vi "server.vi"() -> ()   [LabVIEW 2016]
uses:
  <vilib>/NI/NI JSONRPC Server Framework/Classes/Server/Send Request (Sync).vi
  <vilib>/NI/NI JSONRPC Server Framework/Classes/Server/JSONRPC Server.lvclass
panel:
  in  "stop server":bool
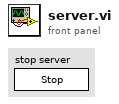
[diagram p1: front panel]
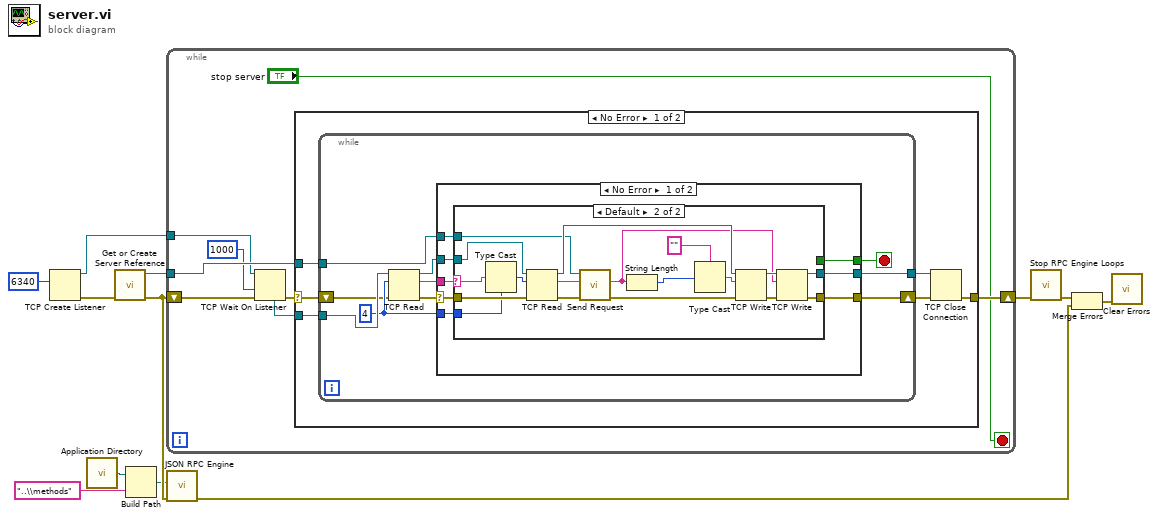
[diagram p0: block diagram]
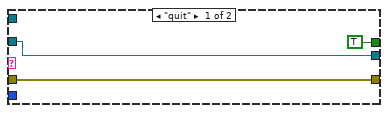
[diagram p2: hidden frame]
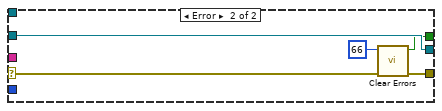
[diagram p3: hidden frame]
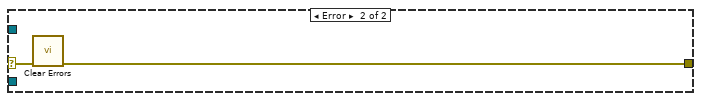
[diagram p4: hidden frame]
diagram:
  n1 = TCP Create Listener(10:u16 6340 ("remote port or service name")) -> (0:w6:errorcluster, 3:w8:refnum<k5>)  [unwired: 4 in, 1 out]
  n2 = call <vilib>:"Application Directory.vi"() -> ("Application Directory"=w3:path)
  n3 = call <vilib>:"Get or Create Server Reference.vi"("error in (no error)"=w6) -> ("error out"=w5:errorcluster, "Server Out"=w12:refnum<class "JSONRPC Server.lvclass">)  [unwired: 9 in]
  n4 = Build Path(base path=w3, name or relative path="..\\methods") -> (appended path=w1:path)
  n5 = while {
    tunnel: w12 -> [w20]
    tunnel: w8 -> [w18]
    shift-right: [w19] -> w11
    shift-left: w5 -> [w16]
    stop <- "stop server" stop-if-true
    n6 = TCP Wait On Listener(8:w16, 9:1000 ("timeout ms (wait forever: -1)"), 11:w18) -> (0:w15:errorcluster, 4:w17:refnum<k5>)  [unwired: 1 in, 3 out]
    n7 = case shown="No Error" w15 {
      selector: w15 -> [w21 w72]
      tunnel: w20 -> [w26 _]
      tunnel: [w25 w71] -> w19
      tunnel: w17 -> [w22 _]
      frame No Error {
        n8 = while {
          tunnel: w26 -> [w36]
          shift-right: [w28] -> w24
          shift-left: w21 -> [w29]
          tunnel: [w35] -> w23
          tunnel: w22 -> [w34]
          stop <- w27 stop-if-true
          w31 = 4 ("bytes to read")
          n9 = TCP Read(connection ID=w34, bytes to read=w31, error in (no error)=w29) -> (connection ID out=w32:refnum<k5>, data out=w33:string, error out=w30:errorcluster)  [unwired: 2 in]
          n10 = case shown="No Error" w30 {
            selector: w30 -> [w44 w68]
            tunnel: w33 -> [w43 _]
            tunnel: w32 -> [w42 w69]
            tunnel: [w41 w69] -> w35
            tunnel: [w40 w70] -> w28
            tunnel: w31 -> [w39 _]
            tunnel: w36 -> [w38 _]
            tunnel: [w37 w66] -> w27
            frame No Error {
              n11 = case shown="Default" w43 {
                selector: w43 -> [_ w64]
                tunnel: w44 -> [w47 w65]
                tunnel: w42 -> [w46 w63]
                tunnel: [w46 w62] -> w41
                tunnel: [w47 w61] -> w40
                tunnel: w39 -> [_ w53]
                tunnel: w38 -> [_ w49]
                tunnel: [TRUE _] -> w37
                frame "quit" {
                }
                frame Default {
                  n12 = Type Cast(type=w53, x=w64) -> (*(type *) &x=w54:i32)
                  n13 = TCP Read(connection ID=w63, bytes to read=w54, error in (no error)=w65) -> (connection ID out=w58:refnum<k5>, data out=w48:string, error out=w52:errorcluster)  [unwired: 2 in]
                  n14 = call-poly <vilib>:"Send Request.vi"("error in (no error)"=w52, "JSON Request String"=w48, "JSONRPC Server in"=w49) -> ("error out"=w51:errorcluster, "JSON Response String"=w50:string)  [unwired: 6 in, 1 out]
                  n15 = String Length(string=w50) -> (length=w57:i32)
                  n16 = Type Cast(type="", x=w57) -> (*(type *) &x=w55:string)
                  n17 = TCP Write(connection ID=w58, data in=w55, error in (no error)=w51) -> (connection ID out=w59:refnum<k5>, error out=w60:errorcluster)  [unwired: 1 in, 1 out]
                  n18 = TCP Write(connection ID=w59, data in=w50, error in (no error)=w60) -> (connection ID out=w62:refnum<k5>, error out=w61:errorcluster)  [unwired: 1 in, 1 out]
                }
              }
            }
            frame Error {
              n19 = call <vilib>:"Clear Errors.vi"("error in (no error)"=w68, "specific error code to clear (0: all)"=66) -> ("error out"=w70:errorcluster, "specific error cleared?"=w66:bool)  [unwired: 4 in]
            }
          }
        }
        n20 = TCP Close Connection(connection ID=w23, error in (no error)=w24) -> (error out=w25:errorcluster)  [unwired: 1 in, 1 out]
      }
      frame Error {
        n21 = call <vilib>:"Clear Errors.vi"("error in (no error)"=w72) -> ("error out"=w71:errorcluster)  [unwired: 5 in, 1 out]
      }
    }
  }
  n22 = call <vilib>:"JSON RPC Engine.vi"("error in (no error)"=w5, "methods directory"=w1) -> ("error out"=w10:errorcluster)  [unwired: 9 in]
  n23 = call <vilib>:"Stop RPC Engine Loops.vi"("error in (no error)"=w11) -> ("error out"=w7:errorcluster)  [unwired: 10 in]
  n24 = Merge Errors(w7, w10) -> (w4:errorcluster)
  n25 = call <vilib>:"Clear Errors.vi"("error in (no error)"=w4) -> ()  [unwired: 5 in, 2 out]
